vi "check_response_parser.vi"(8 "error in (no error)":errorcluster, 11 "response JSON":string) -> (0 "error out":errorcluster, 2 "selector":string, 3 "Response cluster":T1)   [LabVIEW 2015]
uses:
  <vilib>/Utility/error.llb/DialogType.ctl
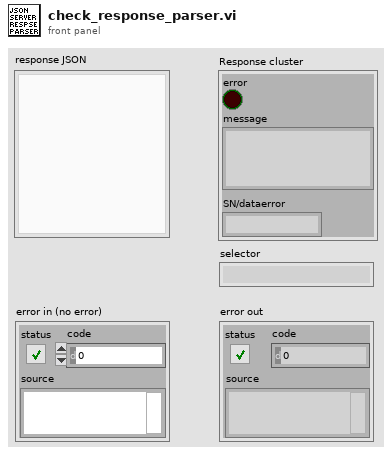
[diagram p1: front panel]
types:
  T1 = cluster{"error":bool, "message":string, "SN/dataerror":string}
  T2 = cluster{"error":bool, "message":string, "serial_number":string}
  T3 = cluster{"error":bool, "message":string, "dataerror":string}
  T4 = typedef "DialogType.ctl" = u16
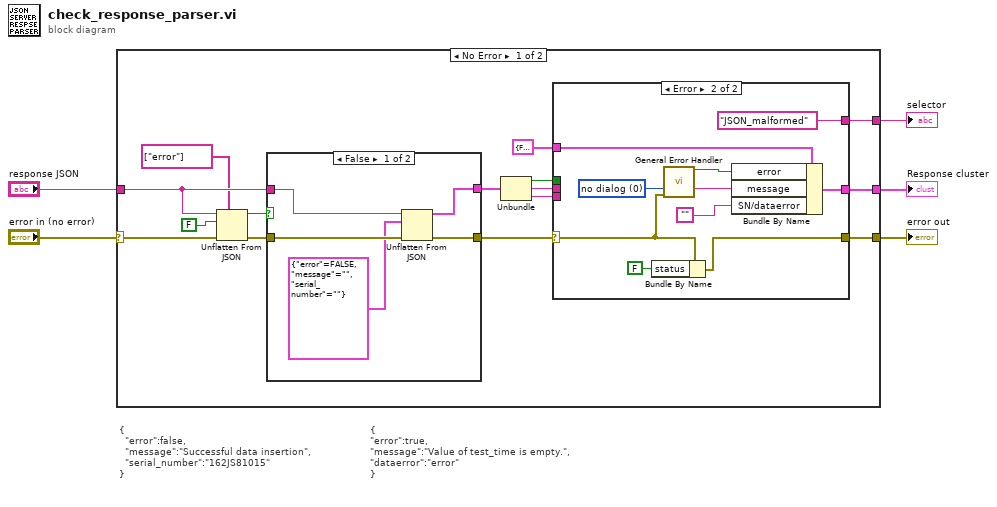
[diagram p0: block diagram]
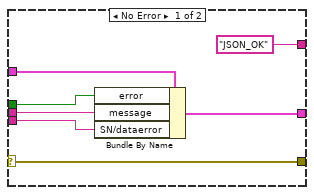
[diagram p2: hidden frame]
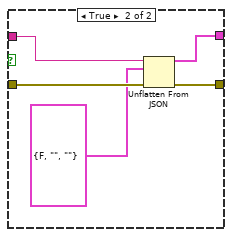
[diagram p3: hidden frame]
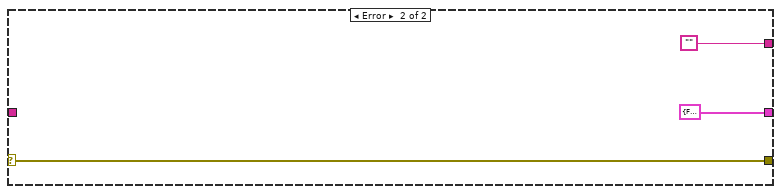
[diagram p4: hidden frame]
diagram:
  # "{\n\"error\":true,\n\"message\":\"Value of test_time is empty.\",\n\"dataerror\":\"error\"\n}"
  # "{\n  \"error\":false,\n  \"message\":\"Successful data insertion\",\n  \"serial_number\":\"162JS81015\"\n}"
  n1 = case shown="No Error" "error in (no error)" {
    selector: "error in (no error)" -> [w19 w50]
    tunnel: "response JSON" -> [w18 _]
    tunnel: [w14 w50] -> w3
    tunnel: [w9 T1 {"error"=FALSE, "message"="", "SN/dataerror"=""}] -> w2
    tunnel: [w6 ""] -> w1
    frame No Error {
      n2 = Unflatten From JSON(path=string[] ["error"], JSON string=w18, type and defaults=FALSE, error in (no error)=w19) -> (value=w16:bool, error out=w17:errorcluster)  [unwired: 3 in]
      n3 = case shown="False" w16 {
        tunnel: w18 -> [w42 w46]
        tunnel: w17 -> [w41 w47]
        tunnel: [w39 w44] -> w15
        tunnel: [w38 w43] -> w13
        frame False {
          n4 = Unflatten From JSON(JSON string=w42, type and defaults=T2 {"error"=FALSE, "message"="", "serial_number"=""}, error in (no error)=w41) -> (value=w38:T2, error out=w39:errorcluster)  [unwired: 4 in]
        }
        frame True {
          n5 = Unflatten From JSON(JSON string=w46, type and defaults=T3 {"error"=FALSE, "message"="", "dataerror"=""}, error in (no error)=w47) -> (value=w43:T3, error out=w44:errorcluster)  [unwired: 4 in]
        }
      }
      n6 = Unbundle(w13) -> ("error"=w12:bool, "message"=w11:string, "dataerror"=w10:string)
      n7 = case shown="Error" w15 {
        selector: w15 -> [w27 w30]
        tunnel: [w27 w37] -> w14
        tunnel: w12 -> [w25 _]
        tunnel: w11 -> [w26 _]
        tunnel: w10 -> [w24 _]
        tunnel: [w23 w35] -> w9
        tunnel: T1 {"error"=FALSE, "message"="", "SN/dataerror"=""} -> [w22 w34]
        tunnel: ["JSON_OK" "JSON_malformed"] -> w6
        frame No Error {
          n8 = Bundle By Name(cluster=w22, "error"=w25, "message"=w26, "SN/dataerror"=w24) -> (w23:T1)
        }
        frame Error {
          w32 = T4 0 items=["no dialog", "OK message", "continue or stop message", "OK message + warnings", "continue/stop + warnings"] ("type of dialog (OK msg:1)")
          n9 = Bundle By Name(cluster=w30, "status"=FALSE) -> (w37:errorcluster)
          n10 = call <vilib>:"General Error Handler.vi"("type of dialog (OK msg:1)"=w32, "error in (no error)"=w30) -> ("error?"=w29:bool, "message"=w31:string)  [unwired: 9 in, 3 out]
          n11 = Bundle By Name(cluster=w34, "error"=w29, "message"=w31, "SN/dataerror"="") -> (w35:T1)
        }
      }
    }
    frame Error {
    }
  }
  "error out" <- w3
  "Response cluster" <- w2
  "selector" <- w1
